vi "Write Repetitions.vi"(8 "error in (no error)":errorcluster, 10 "Repetitions":u32=1 min=1, 11 "Schedule Cell in":refnum<class "Schedule Cell.lvclass">) -> (0 "error out":errorcluster, 3 "Schedule Cell out":refnum<class "Schedule Cell.lvclass">)   [LabVIEW 2020, in "Run Utilities.lvlib" / "Schedule Cell.lvclass"]
uses:
  Schedule Cell.lvclass
  Schedule Cell.lvclass/Schedule Cell.ctl
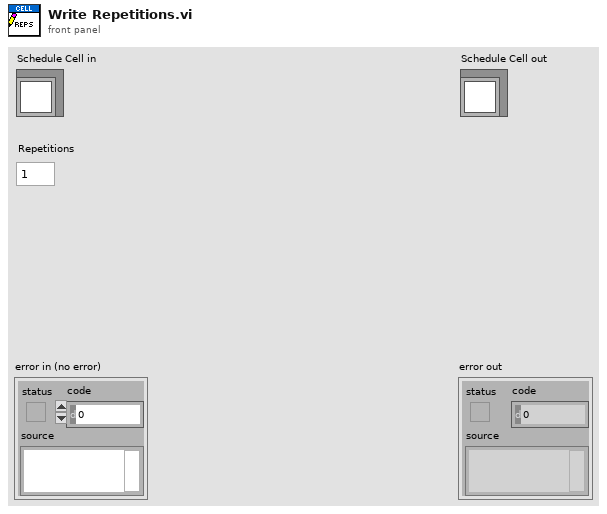
[diagram p1: front panel]
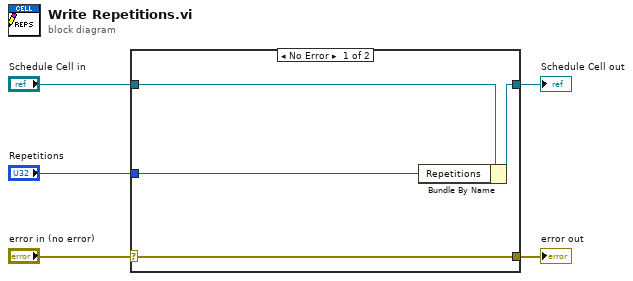
[diagram p0: block diagram]
diagram:
  n1 = case shown="No Error" "error in (no error)" {
    selector: "error in (no error)" -> [w9 w10]
    tunnel: [w9 w10] -> w4
    tunnel: [w7 w11] -> w2
    tunnel: "Schedule Cell in" -> [w8 w11]
    tunnel: "Repetitions" -> [w6 _]
    frame No Error {
      n2 = Bundle By Name(cluster=w8, "Repetitions"=w6) -> (w7:refnum<class "Schedule Cell.lvclass">)
    }
    frame Error {
    }
  }
  "error out" <- w4
  "Schedule Cell out" <- w2
